vi "enumerateStaticDependencies.vi"(8 "error in (no error)":errorcluster, 11 "SMO.A":refnum<class "SMO.A.lvclass">) -> (0 "error out":errorcluster, 2 "Static Dependencies":refnum<class "Dependency.lvclass">[](array[class]), 3 "SMO.A out":refnum<class "SMO.A.lvclass">)   [LabVIEW 2013, in "SMO.A.lvclass"]
uses:
  SMO.A.lvclass
  src/Dependency/Dependency.lvclass
  SMO.B/SMO.B.lvclass
  src/SMO/SMO.lvclass
panel:
  # "For instructions on how to use the JKI State Machine Objects, examples and video tutorials, visit:\nhttp://jki.net/state-machine-objects/\n\nJKI State Machine Objects™\nhttp://jki.net/state-machine-objects/\nCopyright (C) 2005-2015, JKI <info@jki.net>\nALL RIGHTS RESERVED"
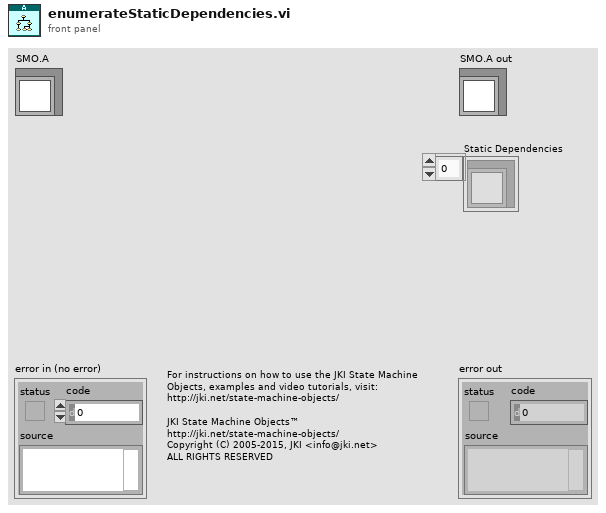
[diagram p1: front panel]
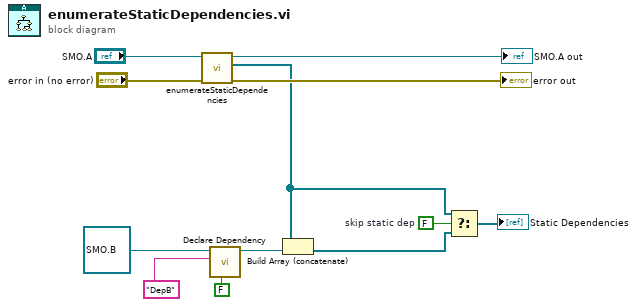
[diagram p0: block diagram]
diagram:
  w4 = FALSE  # skip static dep
  n1 = call-parent "enumerateStaticDependencies.vi"("error in (no error)"="error in (no error)", "SMO"="SMO.A") -> ("error out"=→"error out":errorcluster, "Static Dependencies"=w3:refnum<class "Dependency.lvclass">[], "SMO out"=→"SMO.A out":refnum<class "SMO.A.lvclass">)  [unwired: 7 in]
  n2 = call "Declare Dependency.vi"("Shared Resource (F)"=FALSE, "Name"="DepB", "Type"=refnum<class "SMO.B.lvclass"> refnum ("SMO.B.lvclass")) -> ("Dependency out"=w6:refnum<class "Dependency.lvclass">)  [unwired: 7 in, 1 out]
  n3 = Build Array (concatenate)(w3, w6) -> (w1:refnum<class "Dependency.lvclass">[])
  n4 = Select(t=w3, s=w4, f=w1) -> (s? t:f=→"Static Dependencies":refnum<class "Dependency.lvclass">[])
